vi "Read Payload.vi"(8 "error in (no error)":errorcluster, 11 "uMsg in":refnum<class "uMsg.lvclass">) -> (0 "error out":errorcluster, 2 "uData.lvlib:uData.lvclass":refnum<class "uData.lvclass">, 3 "uMsg out":refnum<class "uMsg.lvclass">)   [LabVIEW 2023, in "uLib.lvlib" / "uMsg.lvclass"]
uses:
  uMsg.lvclass
  uData/uData/uData.lvclass
  uMsg.lvclass/uMsg.ctl
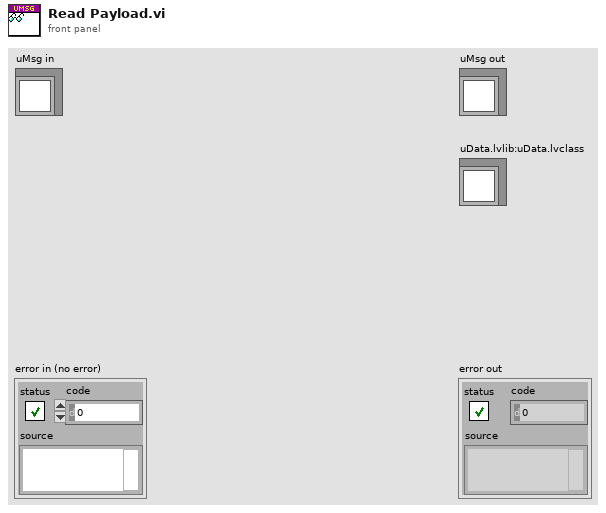
[diagram p1: front panel]
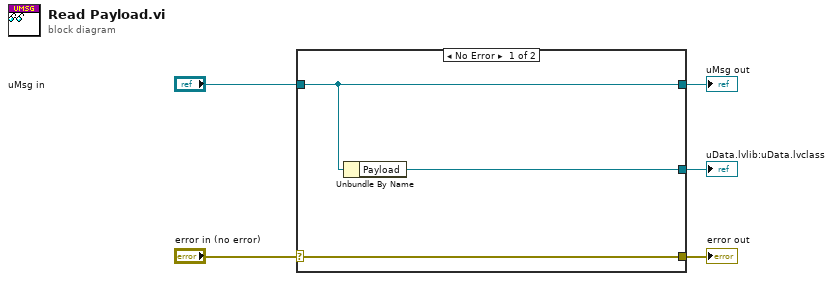
[diagram p0: block diagram]
diagram:
  n1 = case shown="No Error" "error in (no error)" {
    selector: "error in (no error)" -> [w8 w9]
    tunnel: [w8 w9] -> w4
    tunnel: [w7 w10] -> w2
    tunnel: "uMsg in" -> [w7 w10]
    tunnel: [w6 _] -> w1
    frame No Error {
      n2 = Unbundle By Name(w7) -> ("Payload"=w6:refnum<class "uData.lvclass">)
    }
    frame Error {
    }
  }
  "error out" <- w4
  "uMsg out" <- w2
  "uData.lvlib:uData.lvclass" <- w1
